vi "Pre Launch Init.vi"(11 "Optimization in":refnum<class "Optimization.lvclass">) -> (0 "error out":errorcluster, 3 "Optimization out":refnum<class "Optimization.lvclass">)   [LabVIEW 2016, in "Optimization Framework.lvlib" / "Optimization.lvclass"]
doc: "(<B>Filename</B>: Actor Framework.lvlib:Actor.lvclass:Pre Launch Init.vi)\n\nDefines behavior that occurs after the Launch Nested Actor method is invoked but before the actor's Actor Core method begins running.\n\nBy default, this method does nothing. A descendant class may override it to define behavior."
uses:
  Optimization.lvclass
  Controls/Microgrid State Selector.ctl
  Controls/Optimization User Events.ctl
  Controls/Measurement Cluster Energy Storage.ctl
  Controls/3-phase Cluster.ctl
  Controls/Measurement Cluster PV.ctl
  Controls/Measurement Cluster Generator.ctl
  Controls/Measurement Cluster Smart Relay.ctl
  Controls/Schedule Price.ctl
  Controls/Forecast Device Power.ctl
  Controls/PDF Cluster.ctl
  Controls/Optimization Parameters Energy Storage.ctl
  Controls/Device Control Capabilities.ctl
  Controls/Optimization Parameters Generator.ctl
  Master Controller Core/Master Controller/Controls/Current Status.ctl
  Controls/Optimization Parameters Line Configuration.ctl
  Controls/Optimization Line Configuration Enum.ctl
  Optimization.lvclass/Optimization.ctl
  <vilib>/ActorFramework/Actor/Actor.lvclass
  Master Controller Core/Master Controller/Master Controller.lvclass
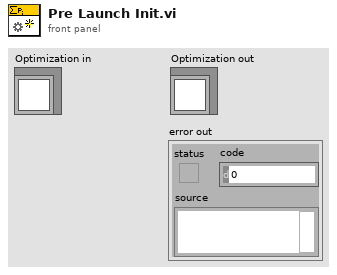
[diagram p1: front panel]
types:
  T1 = typedef "Optimization Framework.lvlib/Optimization.lvclass/Optimization Parameters Line Configuration.ctl" = cluster{"DeviceID":u64, "Line Configuration":T2}
  T2 = typedef "Optimization Framework.lvlib/Optimization.lvclass/Optimization Line Configuration Enum.ctl" = enum8{"Invalid", "L-L", "L-N", "L-G"}
  T3 = typedef "Optimization Framework.lvlib/Optimization.lvclass/Optimization Parameters Generator.ctl" = cluster{"Device ID ":u64, "Bus ID":u16, "Voltage (V)":dbl, "Min Power (kVA)":dbl, "Power Rating (kVA)":dbl, "Ramp Rate (kW/s)":dbl, "Max PF Magnitude (leading)":dbl, "Max PF Magnitude (lagging)":dbl, "Efficiency Curve Power":dbl[], "Efficiency Curve Efficiency":dbl[], "Start-up Time (s)":dbl, "Start-up Cost":dbl, "Fuel Cost":dbl, "Current Status":T4, "Control Capabilities":T5}
  T4 = typedef "Master Controller Core.lvlib/Master Controller.lvclass/Current Status.ctl" = enum8{"Off", "On"}
  T5 = typedef "Optimization Framework.lvlib/Optimization.lvclass/Device Control Capabilities.ctl" = cluster{"VF":bool, "P":bool, "Q":bool, "PF":bool, "PV":bool}
  T6 = typedef "Optimization Framework.lvlib/Optimization.lvclass/Optimization Parameters Energy Storage.ctl" = cluster{"Device ID":u64, "Bus ID":u16, "Voltage (V)":dbl, "Power Rating (kVA)":dbl, "Energy Rating (kWh)":dbl, "Ramp Rate (kW/s)":dbl, "Max Power Factor (leading)":dbl, "Max Power Factor (lagging)":dbl, "Charging Efficiency Curve Power":dbl[], "Charging Efficiency Curve Efficiency":dbl[], "Discharging Efficiency Curve Power":dbl[], "Discharging Efficiency Curve Efficiency":dbl[], "Min SOC(%)":dbl, "Max SOC(%)":dbl, "Start SOC(%)":dbl, "End SOC(%)":dbl, "Control Capabilities":T5}
  T7 = typedef "Optimization Framework.lvlib/Optimization.lvclass/Forecast Device Power.ctl" = cluster{"Device ID":u64, "t0":timestamp, "dt":dbl, "Power Array":dbl[], "Minimum Power Array":dbl[], "Maximum Power Array":dbl[], "PDF Array":T8[]}
  T8 = typedef "Optimization Framework.lvlib/Optimization.lvclass/PDF Cluster.ctl" = cluster{"P0":dbl, "dP":dbl, "Probability Array":dbl[]}
  T9 = typedef "Optimization Framework.lvlib/Optimization.lvclass/Schedule Price.ctl" = cluster{"t0":timestamp, "dt":dbl, "Price Array":dbl[], "Demand Charge":dbl, "Demand Charge Duration":dbl}
  T10 = typedef "Optimization Framework.lvlib/Optimization.lvclass/Measurement Cluster Smart Relay.ctl" = cluster{"Device ID":u64, "Voltage":T11, "Voltage 2":T11, "Current":T11, "Real Power":T11, "Reactive Power":T11}
  T11 = typedef "Optimization Framework.lvlib/Optimization.lvclass/3-phase Cluster.ctl" = cluster{"Phase A":dbl, "Phase B":dbl, "Phase C":dbl}
  T12 = typedef "Optimization Framework.lvlib/Optimization.lvclass/Measurement Cluster Generator.ctl" = cluster{"Device ID":u64, "Voltage":T11, "Current":T11, "Real Power":T11, "Reactive Power":T11}
  T13 = typedef "Optimization Framework.lvlib/Optimization.lvclass/Measurement Cluster PV.ctl" = cluster{"Device ID":u64, "Irradiance":dbl, "Voltage":T11, "Current":T11, "Real Power":T11, "Reactive Power":T11}
  T14 = typedef "Optimization Framework.lvlib/Optimization.lvclass/Measurement Cluster Energy Storage.ctl" = cluster{"Device ID":u64, "SOC":dbl, "Voltage":T11, "Current":T11, "Real Power":T11, "Reactive Power":T11}
  T15 = typedef "Optimization Framework.lvlib/Optimization.lvclass/Optimization User Events.ctl" = cluster{"Microgrid State":refnum<user-event>, "stop":refnum<user-event>}
  T16 = typedef "Optimization Framework.lvlib/Optimization.lvclass/Microgrid State Selector.ctl" = enum16{"Invalid", "Commissioning", "Activation", "Blackstart", "OnGrid", "OffGrid", "Islanding", "Resynchronization", "Shutdown"}
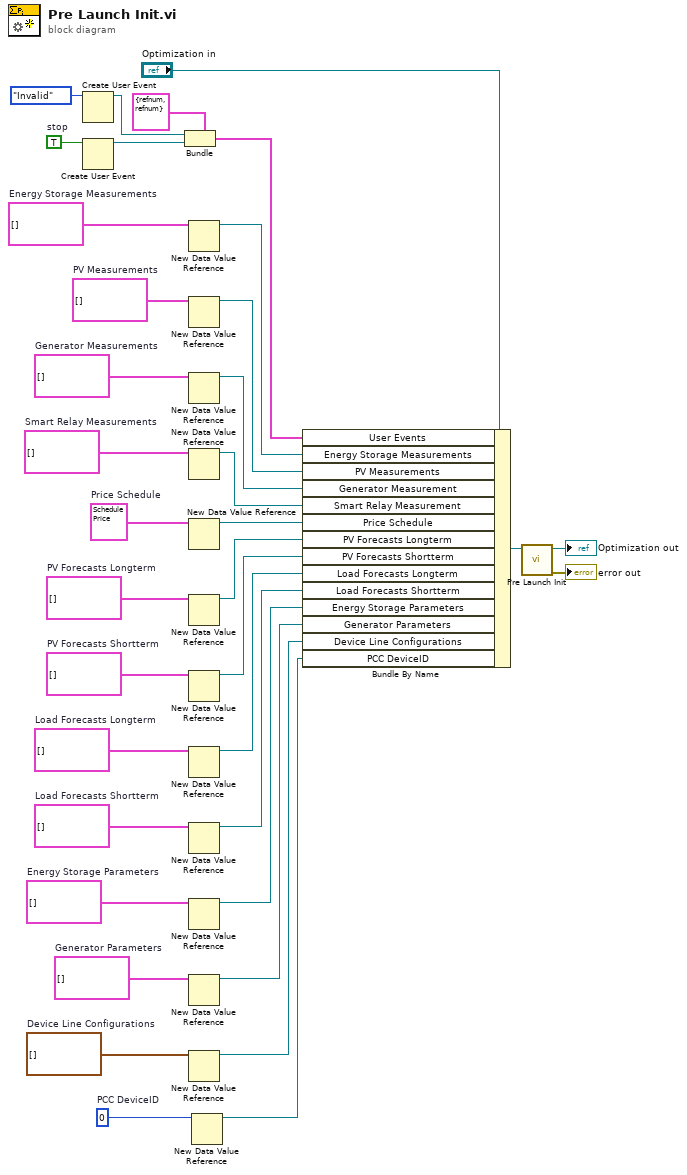
[diagram p0: block diagram]
diagram:
  w14 = u64 0  # PCC DeviceID
  w15 = T1[] []  # Device Line Configurations
  w16 = T3[] []  # Generator Parameters
  w17 = T6[] []  # Energy Storage Parameters
  w18 = T7[] []  # Load Forecasts Shortterm
  w19 = T7[] []  # Load Forecasts Longterm
  w20 = T7[] []  # PV Forecasts Shortterm
  w21 = T7[] []  # PV Forecasts Longterm
  w22 = T9 {"t0"=timestamp(0 s since 1904-01-01), "dt"=0.0, "Price Array"=[], "Demand Charge"=0.0, "Demand Charge Duration"=0.0}  # Price Schedule
  w23 = T10[] []  # Smart Relay Measurements
  w24 = T12[] []  # Generator Measurements
  w25 = T13[] []  # PV Measurements
  w26 = T14[] []  # Energy Storage Measurements
  w29 = TRUE  # stop
  n1 = Create User Event(user event datatype=Microgrid_State_Selector."Invalid" ("Microgrid State")) -> (user event=w30:refnum<user-event>)  [unwired: 1 in, 1 out]
  n2 = Create User Event(user event datatype=w29) -> (user event=w28:refnum<user-event>)  [unwired: 1 in, 1 out]
  n3 = Bundle(cluster=T15 {"Microgrid State"=refnum, "stop"=refnum} ("User Events"), "Microgrid State"=w30, "stop"=w28) -> (w27:T15)
  n4 = New Data Value Reference(data value=w26) -> (data value reference=w12:refnum<data-value>)  [unwired: 1 in, 1 out]
  n5 = New Data Value Reference(data value=w25) -> (data value reference=w8:refnum<data-value>)  [unwired: 1 in, 1 out]
  n6 = New Data Value Reference(data value=w24) -> (data value reference=w11:refnum<data-value>)  [unwired: 1 in, 1 out]
  n7 = New Data Value Reference(data value=w23) -> (data value reference=w9:refnum<data-value>)  [unwired: 1 in, 1 out]
  n8 = New Data Value Reference(data value=w22) -> (data value reference=w7:refnum<data-value>)  [unwired: 1 in, 1 out]
  n9 = New Data Value Reference(data value=w21) -> (data value reference=w5:refnum<data-value>)  [unwired: 1 in, 1 out]
  n10 = New Data Value Reference(data value=w20) -> (data value reference=w3:refnum<data-value>)  [unwired: 1 in, 1 out]
  n11 = New Data Value Reference(data value=w19) -> (data value reference=w1:refnum<data-value>)  [unwired: 1 in, 1 out]
  n12 = New Data Value Reference(data value=w18) -> (data value reference=w2:refnum<data-value>)  [unwired: 1 in, 1 out]
  n13 = New Data Value Reference(data value=w17) -> (data value reference=w6:refnum<data-value>)  [unwired: 1 in, 1 out]
  n14 = New Data Value Reference(data value=w16) -> (data value reference=w10:refnum<data-value>)  [unwired: 1 in, 1 out]
  n15 = New Data Value Reference(data value=w15) -> (data value reference=w13:refnum<data-value>)  [unwired: 1 in, 1 out]
  n16 = New Data Value Reference(data value=w14) -> (data value reference=w4:refnum<data-value>)  [unwired: 1 in, 1 out]
  n17 = Bundle By Name(cluster="Optimization in", "User Events"=w27, "Energy Storage Measurements"=w12, "PV Measurements"=w8, "Generator Measurement"=w11, "Smart Relay Measurement"=w9, "Price Schedule"=w7, "PV Forecasts Longterm"=w5, "PV Forecasts Shortterm"=w3, "Load Forecasts Longterm"=w1, "Load Forecasts Shortterm"=w2, "Energy Storage Parameters"=w6, "Generator Parameters"=w10, "Device Line Configurations"=w13, "PCC DeviceID"=w4) -> (w32:refnum<class "Optimization.lvclass">)
  n18 = call-parent "Pre Launch Init.vi"("Actor in"=w32) -> ("error out"=→"error out":errorcluster, "Actor out"=→"Optimization out":refnum<class "Optimization.lvclass">)  [unwired: 9 in]
